vi "HV_SET.vi"(0 "TCP Network Connection in":refnum<k5>, 2 "DAC_VAL":u32=100, 5 "error in (no error)":errorcluster) -> (14 "TCP Network Connection out":refnum<k5>, 16 "VALUE":u32, 17 "STATUS":u32, 19 "error out":errorcluster)   [LabVIEW 2019]
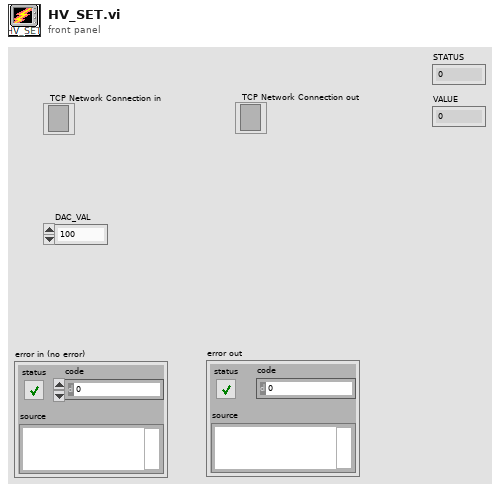
[diagram p1: front panel]
types:
  T1 = enum16{"big-endian, network order", "native, host order", "little-endian"}
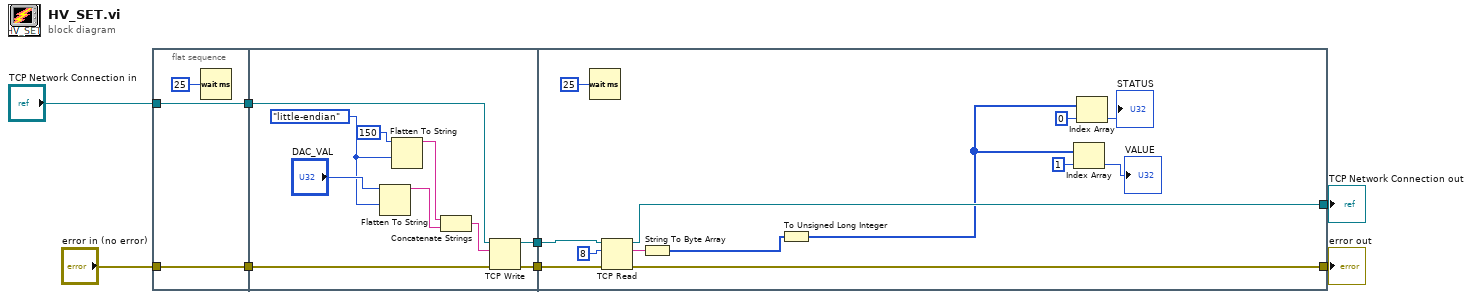
[diagram p0: block diagram]
diagram:
  n1 = flat-sequence {
    tunnel: [w10] -> w4
    tunnel: [w11] -> w3
    tunnel: "error in (no error)" -> [w11]
    tunnel: "TCP Network Connection in" -> [w10]
    tunnel: w4 -> [w21]
    tunnel: w3 -> [w20]
    tunnel: [w19] -> w2
    tunnel: [w18] -> w1
    tunnel: [w31] -> w6
    tunnel: [w32] -> w5
    tunnel: w2 -> [w34]
    tunnel: w1 -> [w33]
    frame #0 {
      n2 = Wait (ms)(milliseconds to wait=u32 25) -> ()  [unwired: 1 out]
    }
    frame #1 {
      w12 = T1."little-endian" ("byte order (0:big-endian, network order)")
      n3 = Flatten To String(anything="DAC_VAL", byte order (0:big-endian, network order)=w12) -> (data string=w17:string)  [unwired: 2 in, 2 out]
      n4 = Flatten To String(anything=u32 150 ("element"), byte order (0:big-endian, network order)=w12) -> (data string=w15:string)  [unwired: 2 in, 2 out]
      n5 = Concatenate Strings(w15, w17) -> (w14:string)
      n6 = TCP Write(connection ID=w21, data in=w14, error in (no error)=w20) -> (connection ID out=w19:refnum<k5>, error out=w18:errorcluster)  [unwired: 1 in, 1 out]
    }
    frame #2 {
      n7 = Wait (ms)(milliseconds to wait=u32 25) -> ()  [unwired: 1 out]
      n8 = TCP Read(connection ID=w34, bytes to read=8, error in (no error)=w33) -> (connection ID out=w32:refnum<k5>, data out=w28:string, error out=w31:errorcluster)  [unwired: 2 in]
      n9 = String To Byte Array(string=w28) -> (unsigned byte array=w27:u8[])
      n10 = To Unsigned Long Integer(number=w27) -> (unsigned 32bit integer=w26:u32[])
      n11 = Index Array(array=w26, index=1) -> (element=→"VALUE":u32)
      n12 = Index Array(array=w26, index=0) -> (element=→"STATUS":u32)
    }
  }
  "error out" <- w6
  "TCP Network Connection out" <- w5
